vi "Status-string.vi"(8 "error in (no error)":errorcluster, 9 "Unit":T1, 10 "Speed":dbl, 11 "Displacement":dbl) -> (0 "error out":errorcluster, 3 "Status string":string)   [LabVIEW 2013, in "PowderDeposition.lvlib" / "Move-Relative.lvclass"]
uses:
  Move-Relative.lvclass
  Motor/Units.ctl
  Motor/Motor.lvclass
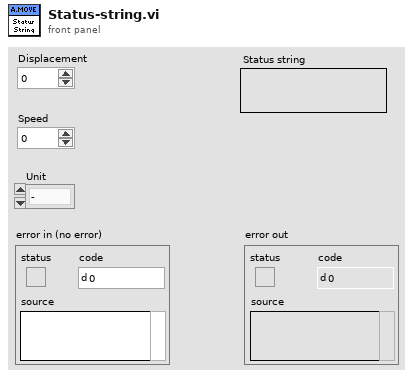
[diagram p1: front panel]
types:
  T1 = typedef "PowderDeposition.lvlib/Motor.lvclass/Units.ctl" = enum16{"-", "mm", "µm", "tr", "V"}
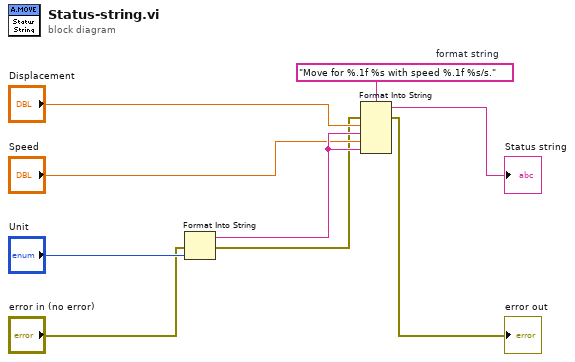
[diagram p0: block diagram]
diagram:
  w8 = "Move for %.1f %s with speed %.1f %s/s."  # format string
  n1 = Format Into String(error in="error in (no error)", "Unit") -> (resulting string=w6:string, error out=w2:errorcluster)  [unwired: 2 in]
  n2 = Format Into String(format string=w8, error in=w2, "Displacement", w6, "Speed", w6) -> (resulting string=→"Status string":string, error out=→"error out":errorcluster)  [unwired: 1 in]
